vi "触发环动报警入队列.vi"(10 "code":i32, 11 "元器件":string) -> ()   [LabVIEW 2016, in "环境动力监测库.lvlib"]
uses:
  Alarm interface/Alarm interface.lvlib
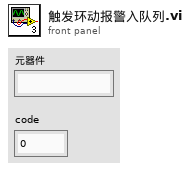
[diagram p1: front panel]
types:
  T1 = typedef "Alarm interface.lvlib/map in.ctl" = cluster{"name":string, "CN":string, "FirmwareVersion":string, "code":string}
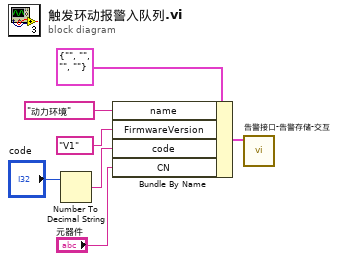
[diagram p0: block diagram]
diagram:
  n1 = Number To Decimal String(number="code") -> (decimal integer string=w4:string)  [unwired: 1 in]
  n2 = Bundle By Name(cluster=T1 {"name"="", "CN"="", "FirmwareVersion"="", "code"=""} ("map in"), "name"="动力环境" ("componentParent"), "FirmwareVersion"="V1" ("equipVersion"), "code"=w4, "CN"="元器件") -> (w2:T1)
  n3 = call "告警接口-告警存储-交互.vi"("map in"=w2) -> ()  [unwired: 10 in, 1 out]
